vi "Display Color Sequence.vi"(1 "Game Data in":T1) -> (0 "Game Data out":T1)   [LabVIEW 2019]
uses:
  Controls/Game Data.ctl
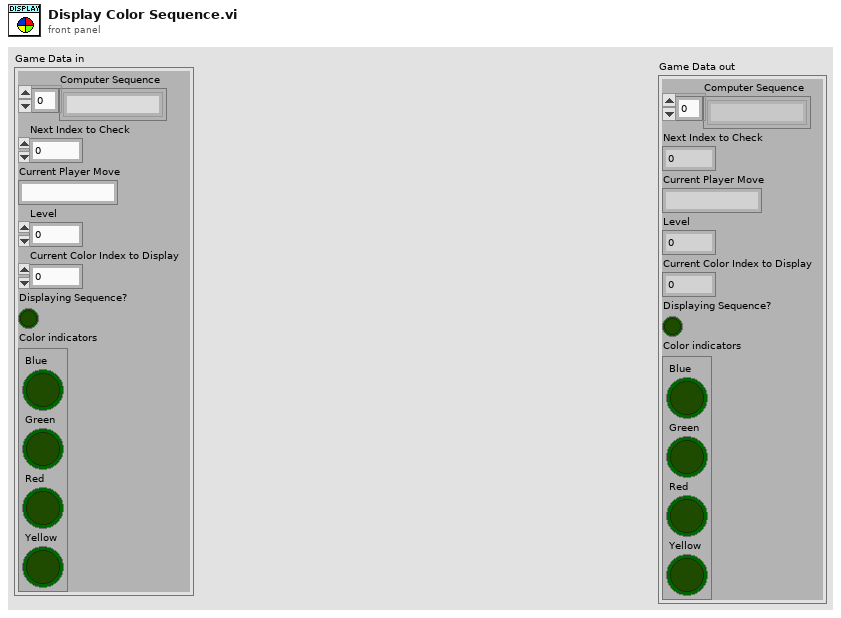
[diagram p1: front panel]
types:
  T1 = typedef "Game Data.ctl" = cluster{"Computer Sequence":string[], "Next Index to Check":i32, "Current Player Move":string, "Level":i32, "Current Color Index to Display":i32, "Displaying Sequence?":bool, "Color indicators":cluster{"Blue":bool, "Green":bool, "Red":bool, "Yellow":bool}}
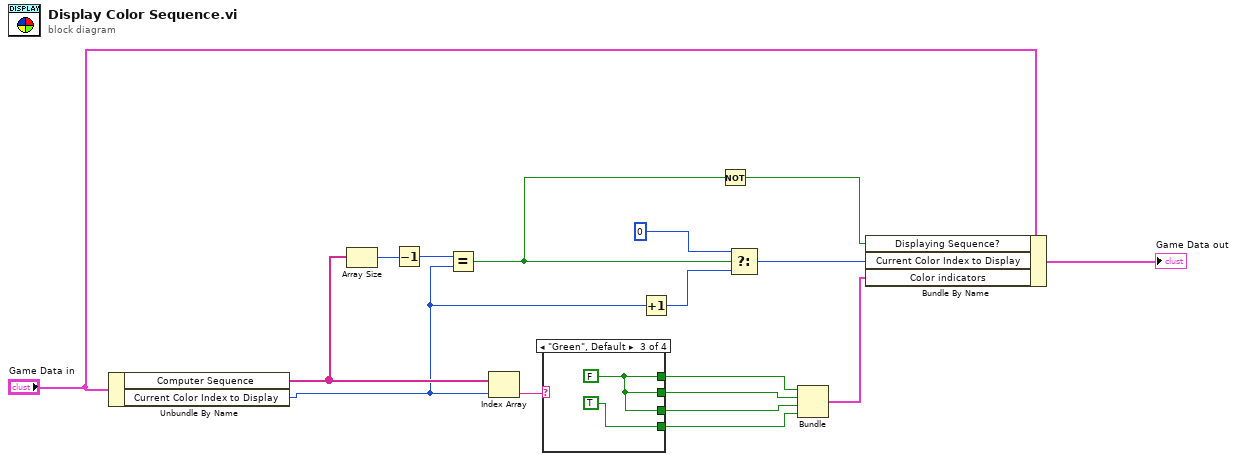
[diagram p0: block diagram]
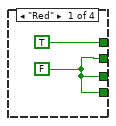
[diagram p2: hidden frame]
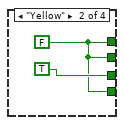
[diagram p3: hidden frame]
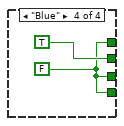
[diagram p4: hidden frame]
diagram:
  n1 = Unbundle By Name("Game Data in") -> ("Computer Sequence"=w14:string[], "Current Color Index to Display"=w5:i32)
  n2 = Array Size(array=w14) -> (size(s)=w13:i32)
  n3 = Decrement(x=w13) -> (x-1=w12:i32)
  n4 = Equal?(x=w12, y=w5) -> (x = y?=w3:bool)
  n5 = Index Array(array=w14, index=w5) -> (element=w15:string)
  n6 = case shown="\"Green\", Default" w15 {
    tunnel: [TRUE w20 w22 w24] -> w11
    tunnel: [w18 w20 w22 TRUE] -> w10
    tunnel: [w18 TRUE w22 w24] -> w9
    tunnel: [w18 w20 TRUE w24] -> w8
    frame "Red" {
      w18 = FALSE
    }
    frame "Yellow" {
      w20 = FALSE
    }
    frame "Green", Default {
      w22 = FALSE
    }
    frame "Blue" {
      w24 = FALSE
    }
  }
  n7 = Increment(x=w5) -> (x+1=w6:i32)
  n8 = Not(x=w3) -> (.not. x?=w2:bool)
  n9 = Select(t=0, s=w3, f=w6) -> (s? t:f=w7:i32)
  n10 = Bundle(w11, w10, w9, w8) -> (w1:cluster{bool, bool, bool, bool})  [unwired: 1 in]
  n11 = Bundle By Name(cluster="Game Data in", "Displaying Sequence?"=w2, "Current Color Index to Display"=w7, "Color indicators"=w1) -> (→"Game Data out":T1)
